vi "Main.vi"() -> ()   [LabVIEW 2014]
uses:
  Tab Panel Data.ctl
  Panel Data.ctl
  Panel Move Modes.ctl
  <vilib>/Utility/miscctls.llb/LVPoint32TypeDef.ctl
  Panel Global Methods.ctl
  <vilib>/Utility/miscctls.llb/LVPositionTypeDef.ctl
  Sub Function/Windows Utilities/WinUtil HWND/Window Style/Get Window GWL_Style.vi
  Sub Function/Windows Utilities/WinUtil HWND/Window Style/Set Window GWL_Style.vi
  Sub Function/Windows Utilities/WinUtil HWND/Get Window HWnd.vi
  Sub Function/Windows Utilities/WinUtil HWND/Get Window Rectangle (hwnd).vi
  <vilib>/Utility/inputDevices.llb/mouseAcquire.vi
  <vilib>/Utility/inputDevices.llb/closeMouse.vi
  <vilib>/Utility/cursorutil.llb/Set Cursor (Icon Pict).vi
  <userlib>/_OpenG.lib/array/array.llb/Conditional Auto-Indexing Tunnel (VI-REF)__ogtk.vi
  Sub Function/Windows Utilities/WinUtil HWND/Window Style/Modify Window Style.vi
  <userlib>/_OpenG.lib/error/error.llb/Build Error Cluster__ogtk.vi
  <vilib>/picture/picture.llb/Draw True-Color Pixmap.vi
panel:
  in  "New Tab":bool
  in  "Tab Control":T1(tab)=enum."Tab 20"
  in  "Move Panel":bool
  in  "Lock Move":bool
  in  "Add":bool
  out "error out":errorcluster
  in  "error in (no error)":errorcluster
  out "2D Picture":picture
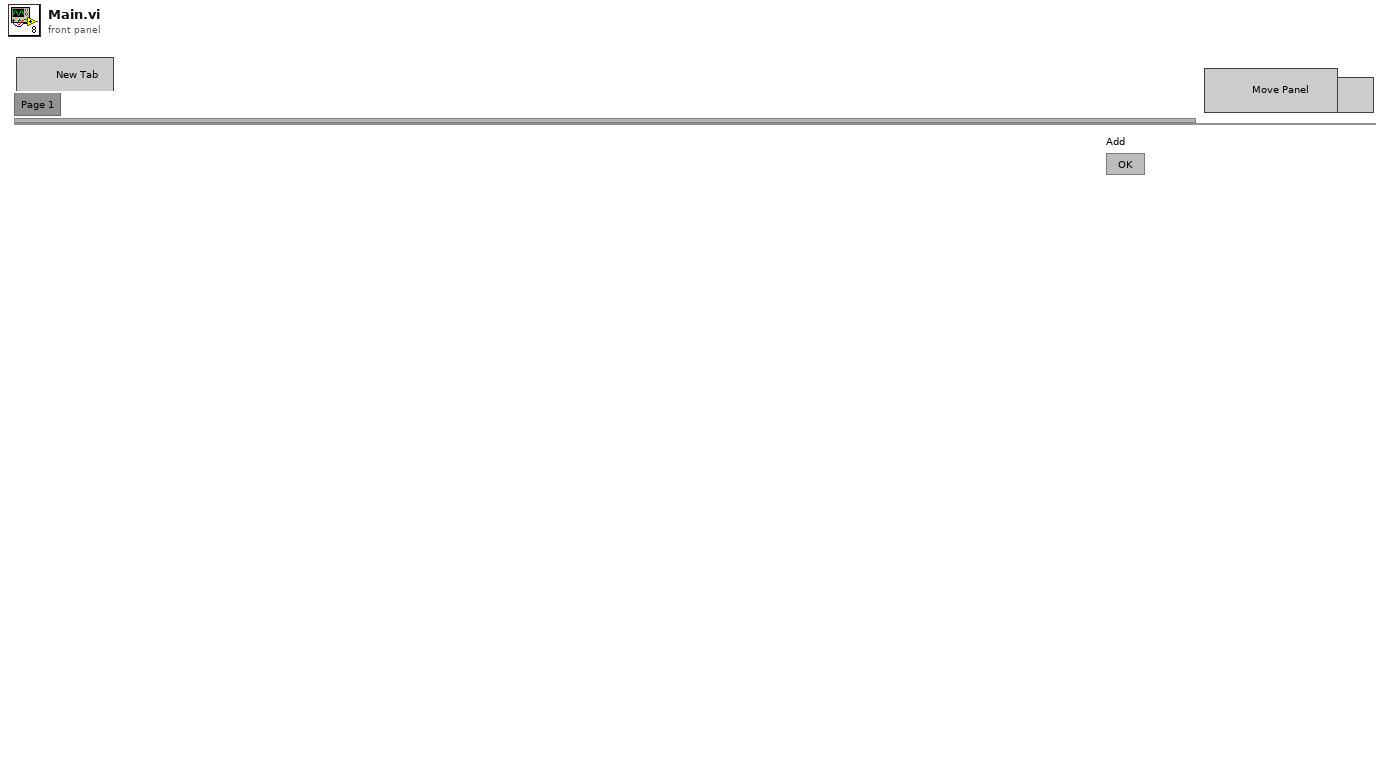
[diagram p1: front panel]
types:
  T1 = enum32{"Tab 1", "Tab 2", "Tab 3", "Tab 4", "Tab 5", "Tab 6", "Tab 7", "Tab 8", "Tab 9", "Tab 10", "Tab 11", "Tab 12", "Tab 13", "Tab 14", "Tab 15", "Tab 16", "Tab 17", "Tab 18", "Tab 19", "Tab 20"}
  T2 = typedef "LVPoint32TypeDef.ctl" = cluster{"Horizontal":i32, "Vertical":i32}
  T3 = typedef "Panel Move Modes.ctl" = enum16{"Move Off", "Move Single", "Move Locked"}
  T4 = typedef "Panel Data.ctl" = cluster{"Panel VI Name":string, "Hwnd":u32, "Collapsed?":bool, "Panel Ref":refnum<vi>, "Events Variant":variant, "Resizeable?":bool, "Un-Dockedable?":bool, "Docked?":bool}
  T5 = typedef "Tab Panel Data.ctl" = cluster{"Tab Name":string, "Tab Visible":bool, "Panel Names":string[]}
  T6 = cluster{"Event Ref":refnum<event-registration>, "New Panel VI Name":string, "Quit Event":refnum<user-event>, "Move Event":refnum<user-event>, "Dock Event":refnum<user-event>, "Panel Move Mode":T3, "Current Panel":T4, "Current Tab":i32, "Previous Tab":i32, "Reposition Offset":cluster{"Left":i16, "Top":i32}, "All Panel Data":T5[], "Parent Hwnd":u32, "Last Mouse Coor Move":T2, "Mouse Down Move":bool, "Handle Resize":bool, "Tab Mouse Coordinates":T2, "Tab Mouse Time":u32, "New Tab Mouse":bool, "Dock Panel In New Tab":bool}
  T7 = typedef "Panel Global Methods.ctl" = enum16{"Read All Panels", "Read Panel Data", "Write Panel Data"}
  T8 = enum8{"Enabled", "Disabled", "Disabled and Grayed Out"}
  T9 = enum32{"Invalid", "Standard", "Closed", "Hidden", "Minimized", "Maximized"}
  T10 = typedef "LVPositionTypeDef.ctl" = cluster{"Left":i32, "Top":i32}
  T11 = cluster{"Width":i16, "Style":enum32{"Solid", "Dash", "Dot", "DashDot", "DashDotDot"}}
  T12 = cluster{"left":i16, "top":i16, "right":i16, "bottom":i16}
  T13 = enum16{"Clear Error And Continue", "Notify User Clear Error", "Clear Error Cleanup"}
  T14 = cluster{"Horizontal":i32, "Vertical":i32, "Scrolling":i32}
  T15 = typedef "lveventtype.ctl" = enum32{"Null", "Timeout", "Annotation Menu Selection", "Annotation Menu Selection?", "App Instance Close", "App Instance Close?", "Autoscale Range Change", "Bookmark Info Change", "Cell Edit", "Cell Edit?", "Cursor Grab", "Cursor Grab?", "Cursor Menu Selection", "Cursor Menu Selection?", "Cursor Move", "Cursor Release", "Data Change", "Direction Change", "Display State Change", "Drag Ended", "Drag Enter", "Drag Leave", "Drag Over", "Drag Source Update", "Drag Starting", "Drag Starting?", "Drop", "Exec State Change", "Key Down", "Key Down?", "Key Repeat", "Key Repeat?", "Key Up", "Listbox Double Click", "Menu Activation?", "Menu Selection (App)", "Menu Selection? (App)", "Menu Selection (User)", "Mouse Down", "Mouse Down?", "Mouse Enter", "Mouse Leave", "Mouse Move", "Mouse Up", "Mouse Wheel", "NI Security User Change (App)", "Pane Size", "Panel Close", "Panel Close?", "Panel Resize", "Plot Attribute Change", "Scale Range Change", "Shortcut Menu Activation?", "Shortcut Menu Selection (App)", "Shortcut Menu Selection? (App)", "Shortcut Menu Selection (User)", "Tree Double Click", "Tree Drag", "Tree Drag?", "Tree Drop", "Tree Drop?", "Tree Item Close", "Tree Item Close?", "Tree Item Open", "Tree Item Open?", "User Event", "Value Change"}
  T16 = typedef "LVRectTypeDef.ctl" = cluster{"Left":i16, "Top":i16, "Right":i16, "Bottom":i16}
  T17 = typedef "LVBoundsTypeDef.ctl" = cluster{"Width":u32, "Height":u32}
  T18 = typedef "Window Rectangle (hwnd).ctl" = cluster{"left":i16, "top":i16, "right":i16, "bottom":i16}
  T19 = typedef "LVPointTypeDef.ctl" = cluster{"Horizontal":i16, "Vertical":i16}
  T20 = typedef "imagedata.ctl" = cluster{"image type":i32, "image depth":i32, "image":u8[], "mask":u8[], "colors":u32[], "Rectangle":cluster{"left":i16, "top":i16, "right":i16, "bottom":i16}}
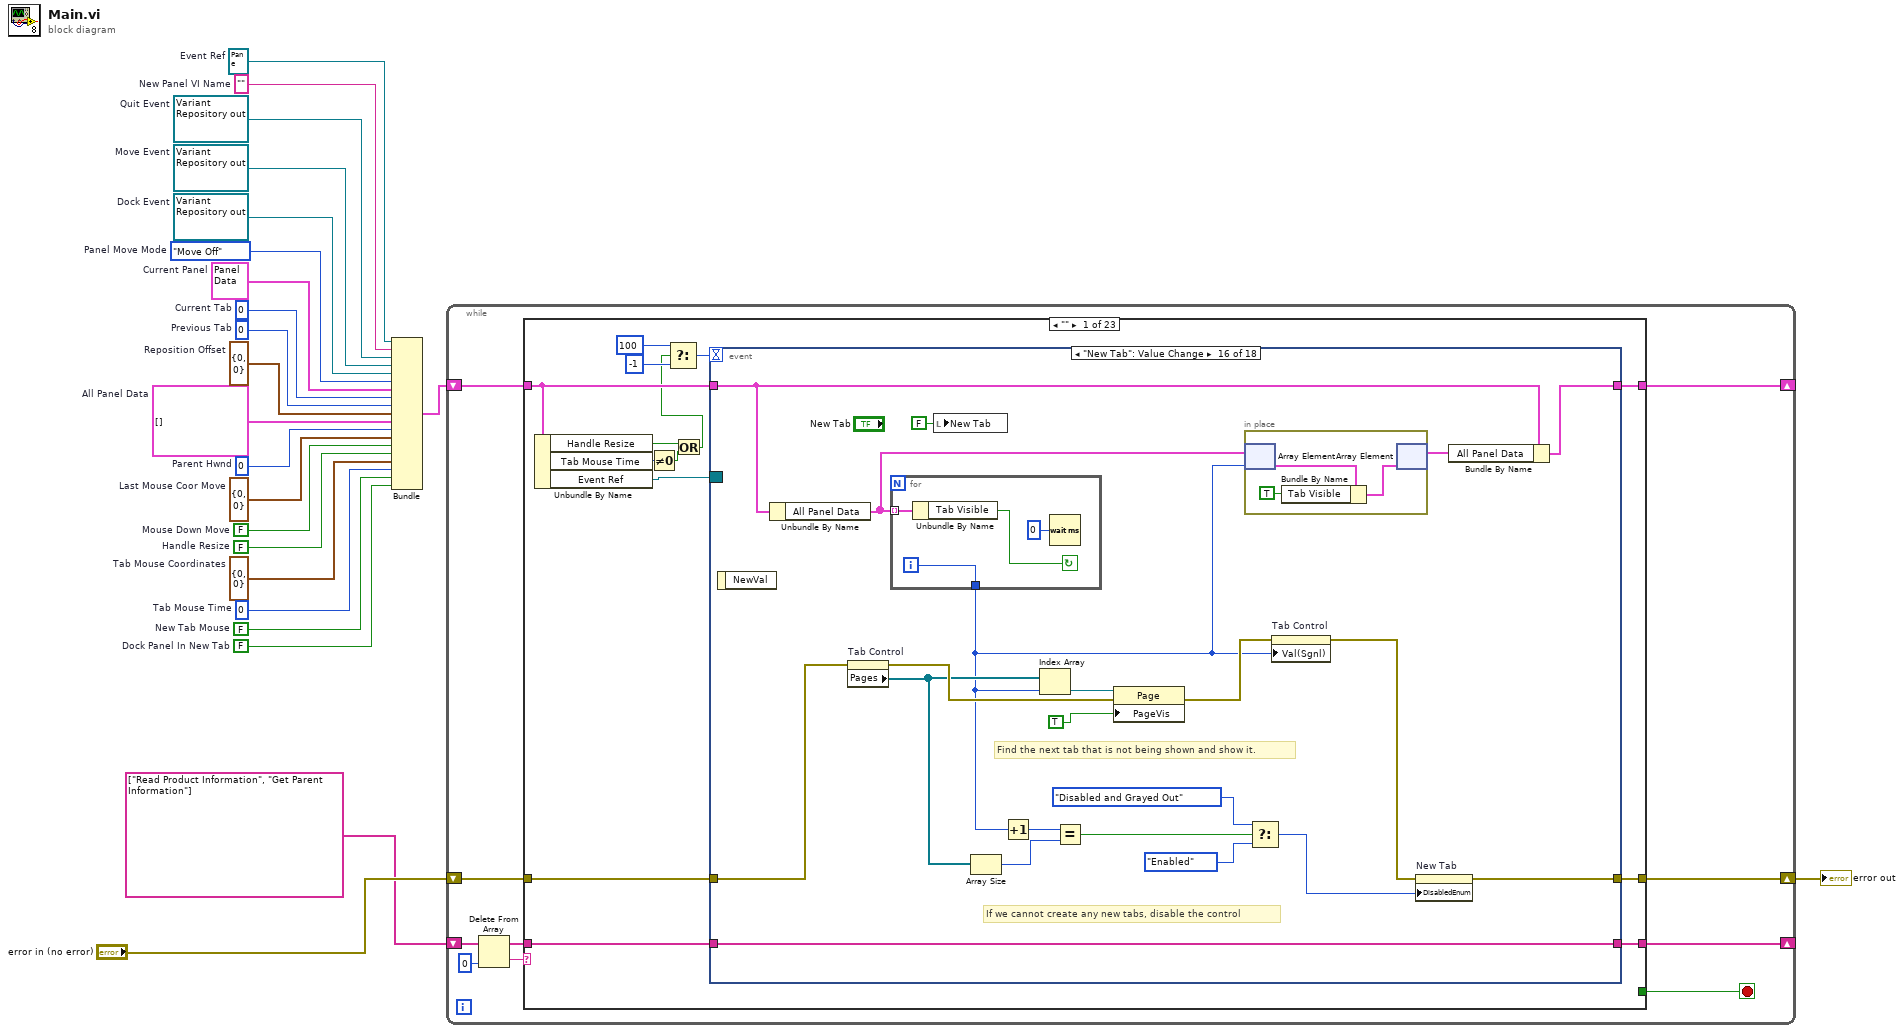
[diagram p0: block diagram]
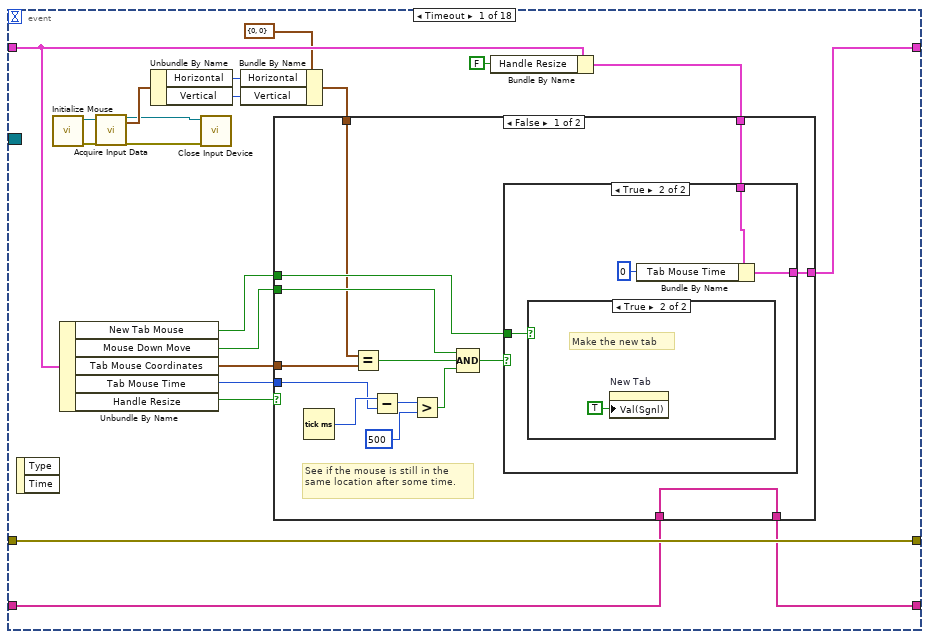
[diagram p2: hidden frame]
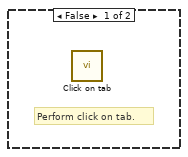
[diagram p4: hidden frame]
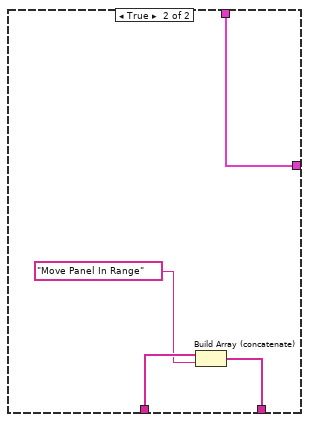
[diagram p5: hidden frame]
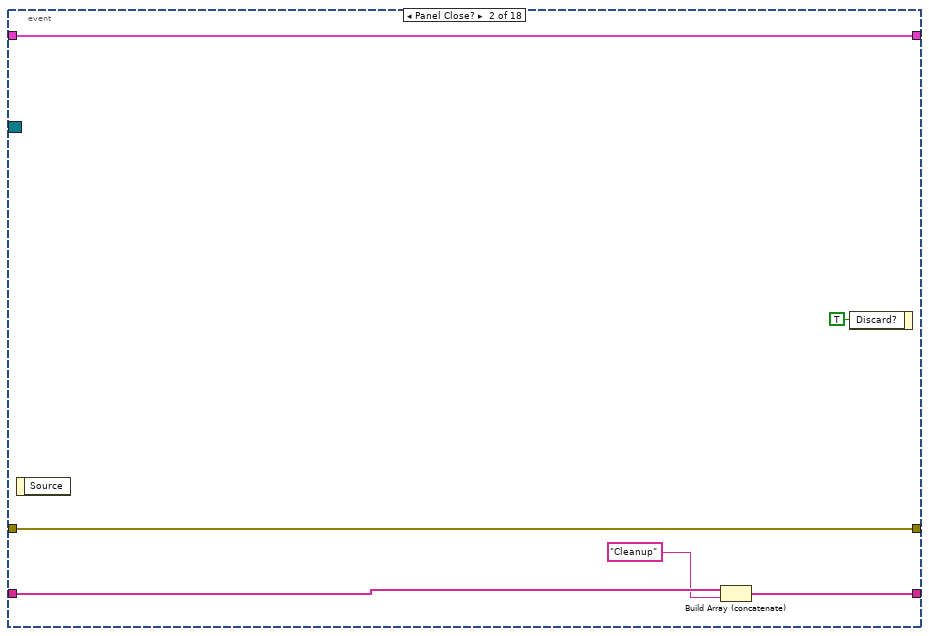
[diagram p6: hidden frame]
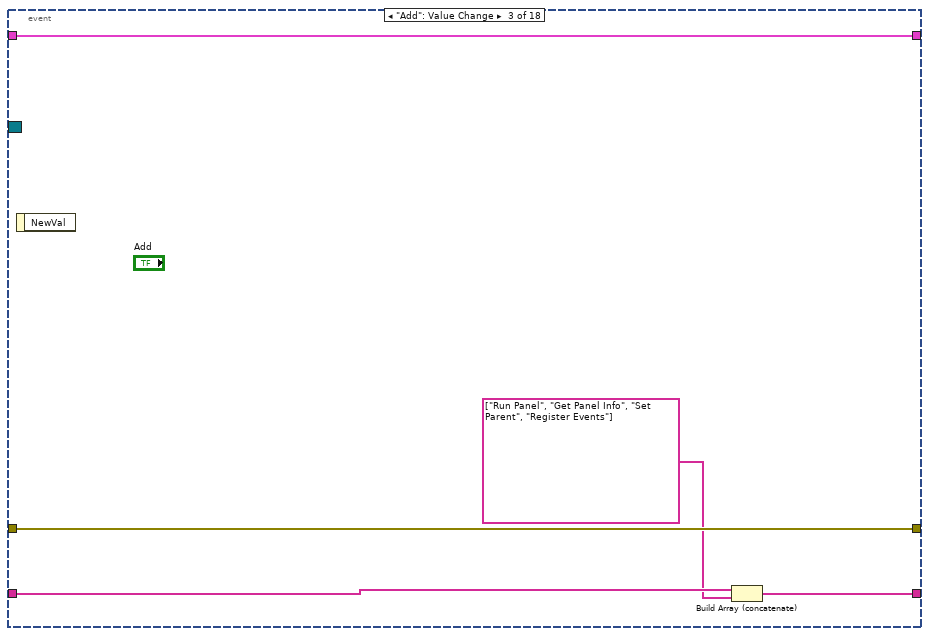
[diagram p7: hidden frame]
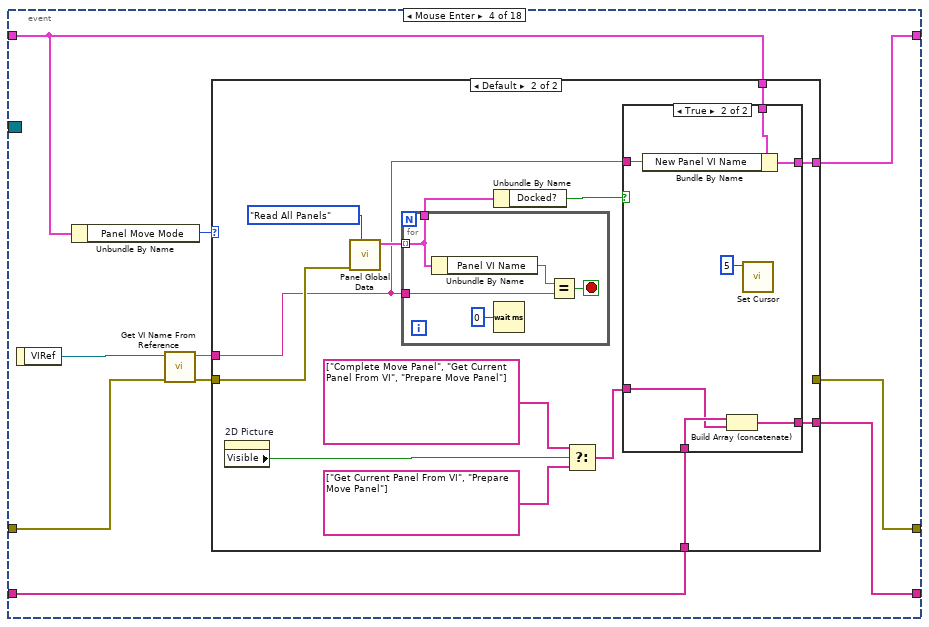
[diagram p8: hidden frame]
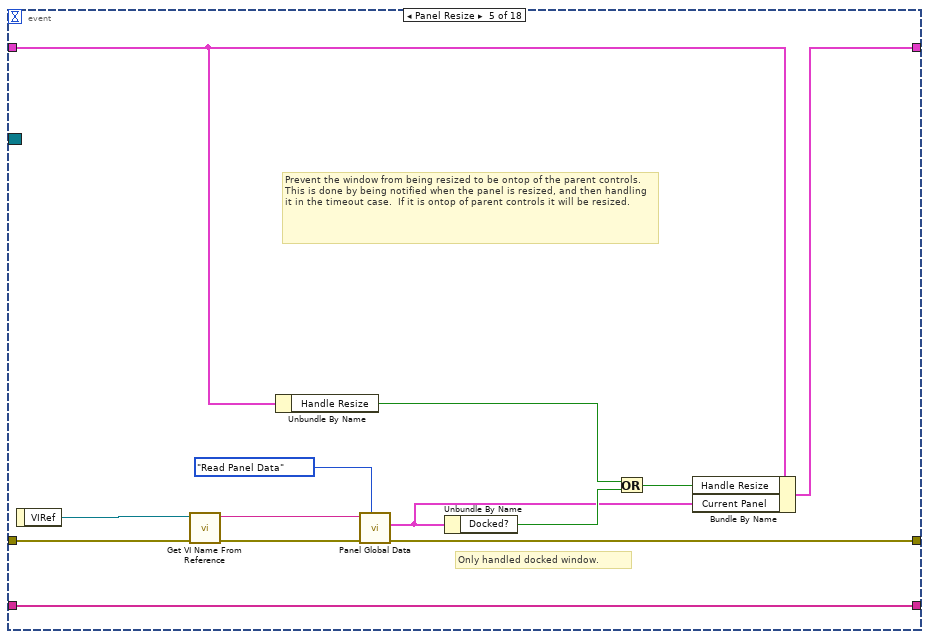
[diagram p11: hidden frame]
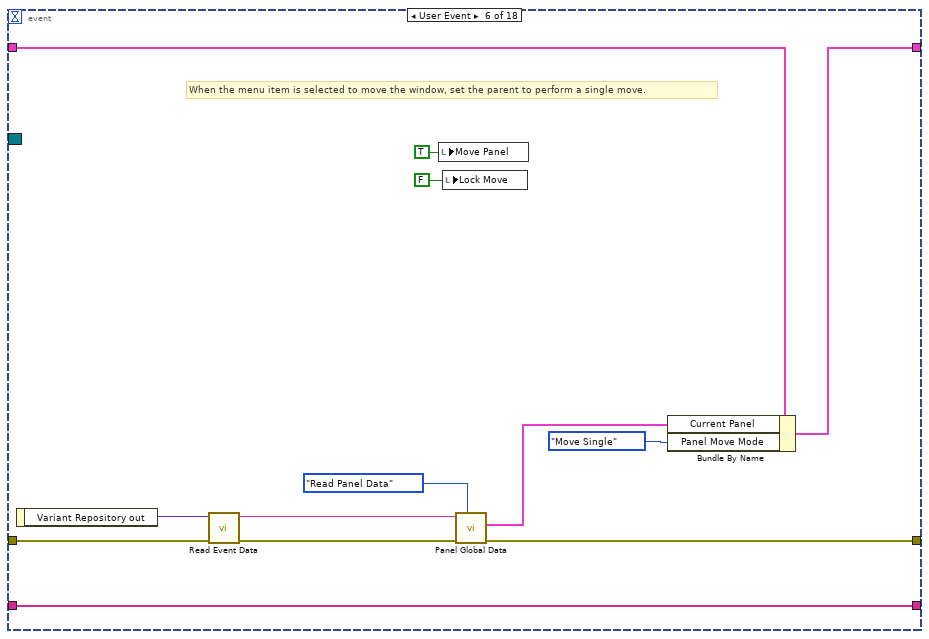
[diagram p12: hidden frame]
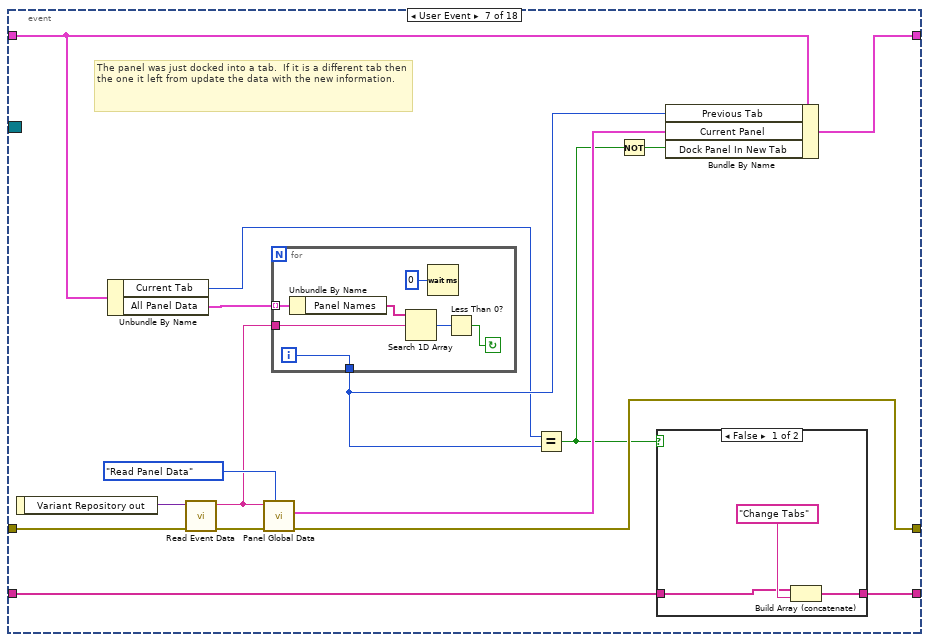
[diagram p13: hidden frame]
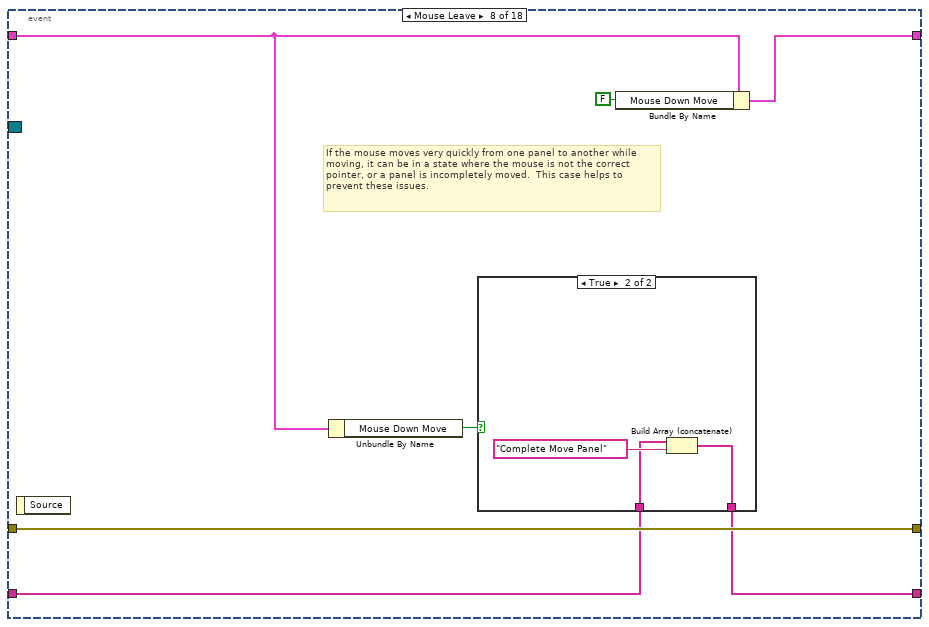
[diagram p15: hidden frame]
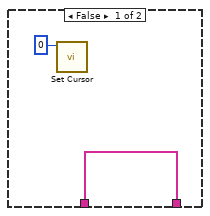
[diagram p16: hidden frame]
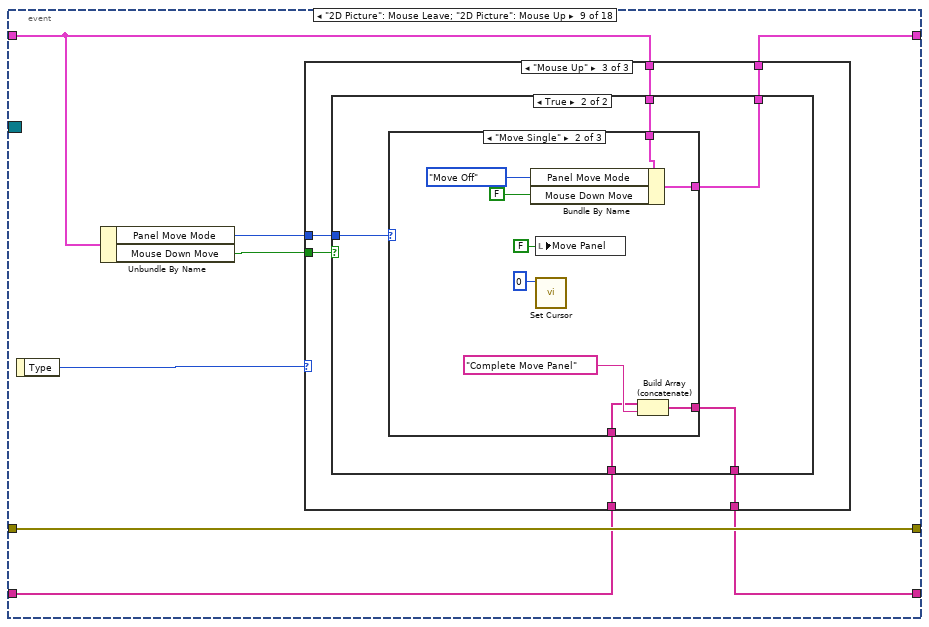
[diagram p17: hidden frame]
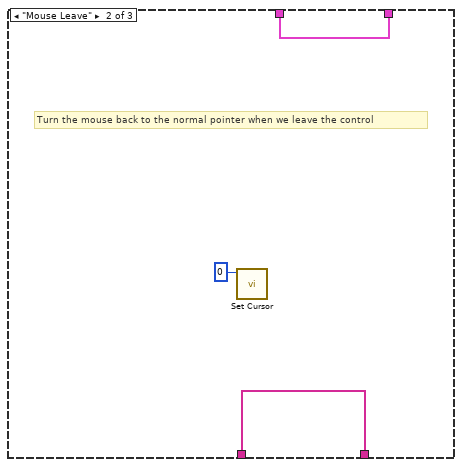
[diagram p19: hidden frame]
diagram:
  w3 = refnum<event-registration> refnum  # Event Ref
  w4 = refnum<user-event> refnum  # Quit Event
  w5 = FALSE  # Dock Panel In New Tab
  w6 = refnum<user-event> refnum  # Dock Event
  w7 = ""  # New Panel VI Name
  w8 = 0  # Previous Tab
  w9 = FALSE  # New Tab Mouse
  w10 = u32 0  # Tab Mouse Time
  w11 = T2 {"Horizontal"=0, "Vertical"=0}  # Tab Mouse Coordinates
  w12 = FALSE  # Handle Resize
  w13 = refnum<user-event> refnum  # Move Event
  w14 = FALSE  # Mouse Down Move
  w15 = T2 {"Horizontal"=0, "Vertical"=0}  # Last Mouse Coor Move
  w16 = u32 0  # Parent Hwnd
  w19 = Panel_Move_Modes."Move Off"  # Panel Move Mode
  w20 = T4 {"Panel VI Name"="", "Hwnd"=0, "Collapsed?"=FALSE, "Panel Ref"=refnum, "Events Variant"=variant, "Resizeable?"=FALSE, "Un-Dockedable?"=FALSE, "Docked?"=FALSE}  # Current Panel
  w21 = 0  # Current Tab
  w17 = T5[] []  # All Panel Data
  w18 = cluster{"Left":i16, "Top":i32} {"Left"=0, "Top"=0}  # Reposition Offset
  n1 = Bundle("Event Ref"=w3, "New Panel VI Name"=w7, "Quit Event"=w4, "Move Event"=w13, "Dock Event"=w6, "Panel Move Mode"=w19, "Current Panel"=w20, "Current Tab"=w21, "Previous Tab"=w8, "Reposition Offset"=w18, "All Panel Data"=w17, "Parent Hwnd"=w16, "Last Mouse Coor Move"=w15, "Mouse Down Move"=w14, "Handle Resize"=w12, "Tab Mouse Coordinates"=w11, "Tab Mouse Time"=w10, "New Tab Mouse"=w9, "Dock Panel In New Tab"=w5) -> (w23:T6)  [unwired: 1 in]
  n2 = while {
    shift-right: [w24] -> _
    shift-left: string[] ["Read Product Information", "Get Parent Information"] ("Initialized States") -> [w27]
    shift-right: [w29] -> w1
    shift-left: "error in (no error)" -> [w33]
    shift-right: [w31] -> _
    shift-left: w23 -> [w32]
    stop <- w30 stop-if-true
    n3 = Delete From Array(array=w27, index=0) -> (deleted portion=w25:string, array with subset deleted=w26:string[])  [unwired: 1 in]
    n4 = case "State Machine" shown="\"\"" w25 {
      selector: w25 -> [_ _ _ _ _ _ _ _ _ _ _ _ w592 _ _ _ _ w731 _ _ _ _ _]
      tunnel: w26 -> [w47 w402 w406 w447 w486 w506 w528 w555 w558 w561 w564 w573 w606 w656 w678 w709 w711 w735 w738 w741 w758 w771 w775]
      tunnel: [w43 w402 w406 w447 w486 w506 w528 w555 w558 w561 w564 w573 w606 w656 w678 w709 w712 w735 w738 w739 w758 w771 w775] -> w24
      tunnel: [w44 w400 w405 w423 w482 w497 w521 w537 w556 w559 w563 w565 w579 w651 w658 w708 w713 w728 w737 w743 w746 w769 w772] -> w29
      tunnel: w33 -> [w45 w400 w405 w417 w470 w494 w515 w542 w556 w559 w563 w566 w580 w650 w663 w708 w714 w729 w737 w743 w752 w770 w772]
      tunnel: w32 -> [w42 w401 w403 w440 w484 w502 w527 w549 w557 w560 w562 w570 w591 w652 w667 w707 w715 w734 w736 w742 w757 w768 w774]
      tunnel: [w46 w401 w403 w443 w485 w503 w522 w541 w557 w560 w562 w568 w591 w652 w662 w707 w715 w734 w736 w742 w757 w768 w774] -> w31
      tunnel: [_ _ _ _ _ _ _ _ _ _ _ _ _ _ _ _ _ _ _ _ _ _ TRUE] -> w30
      frame "" {
        n5 = Unbundle By Name(w42) -> ("Handle Resize"=w35:bool, "Tab Mouse Time"=w37:u32, "Event Ref"=w41:refnum<event-registration>)
        n6 = Not Equal To 0?(x=w37) -> (x != 0?=w36:bool)
        n7 = Or(x=w35, y=w36) -> (x .or. y?=w34:bool)
        n8 = Select(t=100, s=w34, f=-1) -> (s? t:f=w38:i32)
        n9 = event shown="[15] \"New Tab\": Value Change" {
          selector: w41 -> [_ _ _ _ _ _ _ _ _ _ _ _ _ _ _ _ _ _]
          dyn-events: _ -> [_ _ _ _ _ _ _ _ _ _ _ _ _ _ _ _ _ _]
          timeout: w38 -> [_ _ _ _ _ _ _ _ _ _ _ _ _ _ _ _ _ _]
          tunnel: w42 -> [w66 w96 w103 w110 w147 w170 w181 w201 w213 w257 w263 w276 w283 w325 w333 w353 w368 w372]
          tunnel: w47 -> [w67 w95 w101 w108 w157 w163 w186 w203 w215 w256 w269 w278 w281 w324 w327 w354 w366 w374]
          tunnel: [w59 w96 w103 w109 w156 w168 w183 w199 w212 w257 w262 w275 w290 w323 w331 w348 w368 w371] -> w46
          tunnel: w45 -> [w68 w97 w102 w105 w150 w160 w171 w204 w217 w254 w259 w279 w291 w309 w332 w345 w367 w375]
          tunnel: [w68 w97 w102 w104 w149 w162 w177 w204 w217 w253 w258 w279 w291 w308 w332 w338 w367 w375] -> w44
          tunnel: [w64 w93 w99 w107 w157 w163 w184 w202 w214 w256 w269 w278 w280 w324 w326 w354 w366 w374] -> w43
          event Timeout {
            n10 = event-data() -> ()  [unwired: 1 in, 2 out]
            n11 = call <vilib>:"Initialize Mouse.vi"() -> ("error out"=w52:errorcluster, "device ID"=w49:refnum<k1>)  [unwired: 10 in]
            n12 = Unbundle By Name(w66) -> ("New Tab Mouse"=w57:bool, "Mouse Down Move"=w58:bool, "Tab Mouse Coordinates"=w62:T2, "Tab Mouse Time"=w61:u32, "Handle Resize"=w63:bool)
            n13 = call-poly <vilib>:"Acquire Input Data.vi"("device ID"=w49, "error in (no error)"=w52) -> ("device ID"=w50:refnum<k1>, "axis info"=w53:T14, "error out"=w51:errorcluster)  [unwired: 14 in, 1 out]
            n14 = Unbundle By Name(w53) -> ("Horizontal"=w55:i32, "Vertical"=w56:i32)
            n15 = call-poly <vilib>:"Close Input Device.vi"("error in (no error)"=w51, "device ID"=w50) -> ()  [unwired: 8 in, 1 out]
            n16 = Bundle By Name(cluster=cluster{"Horizontal":i32, "Vertical":i32} {"Horizontal"=0, "Vertical"=0} ("Mouse Position"), "Horizontal"=w55, "Vertical"=w56) -> (w48:cluster{"Horizontal":i32, "Vertical":i32})
            n17 = Bundle By Name(cluster=w66, "Handle Resize"=FALSE) -> (w60:T6)
            n18 = case shown="False" w63 {
              tunnel: w67 -> [w72 w91]
              tunnel: [w72 w89] -> w64
              tunnel: w62 -> [w82 _]
              tunnel: w61 -> [w80 _]
              tunnel: w60 -> [w74 w92]
              tunnel: [w73 w92] -> w59
              tunnel: w58 -> [w71 _]
              tunnel: w57 -> [w70 _]
              tunnel: w48 -> [w69 _]
              frame False {
                # "See if the mouse is still in the same location after some time."
                n19 = Tick Count (ms)() -> (millisecond timer value=w81:u32)
                n20 = Equal?(x=w69, y=w82) -> (x = y?=w77:bool)
                n21 = Subtract(x=w81, y=w80) -> (x-y=w79:u32)
                n22 = Greater?(x=w79, y=u32 500) -> (0:w76:bool)
                n23 = Compound Arithmetic op=AND(w71, w77, w76) -> (w75:bool)
                n24 = case shown="True" w75 {
                  tunnel: w74 -> [w83 w87]
                  tunnel: [w83 w85] -> w73
                  tunnel: w70 -> [_ w84]
                  frame False {
                  }
                  frame True {
                    n25 = case shown="True" w84 {
                      frame False {
                        # "Perform click on tab."
                        n26 = call "Click on tab.vi"() -> ()  [unwired: 11 in, 1 out]
                      }
                      frame True {
                        # "Make the new tab"
                        n27 = property on="New Tab" class="Bool (strict)"("Val(Sgnl)"=TRUE ("Value (Signaling)")) -> ()  [unwired: 2 in, 2 out]
                      }
                    }
                    n28 = Bundle By Name(cluster=w87, "Tab Mouse Time"=u32 0) -> (w85:T6)
                  }
                }
              }
              frame True {
                n29 = Build Array (concatenate)(w91, "Move Panel In Range" ("String")) -> (w89:string[])
              }
            }
          }
          event Panel Close? {
            n30 = event-data() -> ()  [unwired: 1 in, 1 out]
            n31 = Build Array (concatenate)(w95, "Cleanup" ("Panel Close Event")) -> (w93:string[])
            n32 = event-data("Discard?"=TRUE) -> ()  [unwired: 1 in, 1 out]
          }
          event "Add": Value Change {
            n33 = event-data() -> ()  [unwired: 1 in, 1 out]
            n34 = Build Array (concatenate)(w101, string[] ["Run Panel", "Get Panel Info", "Set Parent", "Register Events"] ("Elements to Add")) -> (w99:string[])
          }
          event Mouse Enter {
            n35 = event-data() -> ("VIRef"=w112:refnum<vi>)  [unwired: 1 in]
            n36 = Unbundle By Name(w110) -> ("Panel Move Mode"=w113:T3)
            n37 = call "Get VI Name From Reference.vi"("error in (no error)"=w105, "VI Ref"=w112) -> ("error out"=w106:errorcluster, "VI Name"=w111:string)  [unwired: 8 in]
            n38 = case shown="Default" w113 {
              tunnel: w111 -> [_ w121]
              tunnel: w110 -> [w116 w125]
              tunnel: [w116 w124] -> w109
              tunnel: w108 -> [w115 w130]
              tunnel: [w115 w129] -> w107
              tunnel: w106 -> [w114 w122]
              tunnel: [w114 _] -> w104
              frame "Move Off" {
              }
              frame Default {
                n39 = property on="2D Picture" class="Pict"() -> ("Visible"=w117:bool)  [unwired: 2 in, 2 out]
                n40 = call "Panel Global Data.vi"("Method (Read All)"=Panel_Global_Methods."Read All Panels", "error in (no error)"=w122) -> ("All Panel Data"=w127:T4[])  [unwired: 6 in, 3 out]
                n41 = for {
                  tunnel: w121 -> [w143]
                  tunnel: [w140] -> w123
                  tunnel: w127 -> [w140] mode=indexing
                  stop <- w142 stop-if-true
                  n42 = Unbundle By Name(w140) -> ("Panel VI Name"=w144:string)
                  n43 = Wait (ms)(milliseconds to wait=u32 0) -> ()  [unwired: 1 out]
                  n44 = Equal?(x=w144, y=w143) -> (x = y?=w142:bool)
                }
                n45 = Unbundle By Name(w123) -> ("Docked?"=w126:bool)
                n46 = Select(t=string[] ["Complete Move Panel", "Get Current Panel From VI", "Prepare Move Panel"], s=w117, f=string[] ["Get Current Panel From VI", "Prepare Move Panel"]) -> (s? t:f=w118:string[])
                n47 = case shown="True" w126 {
                  tunnel: w130 -> [w132 w135]
                  tunnel: [w132 w133] -> w129
                  tunnel: w125 -> [w131 w138]
                  tunnel: [w131 w137] -> w124
                  tunnel: w118 -> [_ w134]
                  tunnel: w121 -> [_ w136]
                  frame False {
                  }
                  frame True {
                    n48 = Bundle By Name(cluster=w138, "New Panel VI Name"=w136) -> (w137:T6)
                    n49 = Build Array (concatenate)(w135, w134) -> (w133:string[])
                    n50 = call-poly <vilib>:"Set Cursor.vi"("icon"=u16 5) -> ()  [unwired: 9 in, 2 out]
                  }
                }
              }
            }
          }
          event Panel Resize {
            # "Only handled docked window."
            # "Prevent the window from being resized to be ontop of the parent controls.  This is done by being notified when the panel is resized, and then handling it in the timeout case.  If it is ontop of parent controls it will be resized."
            n51 = event-data() -> ("VIRef"=w152:refnum<vi>)  [unwired: 1 in]
            n52 = call "Get VI Name From Reference.vi"("error in (no error)"=w150, "VI Ref"=w152) -> ("error out"=w153:errorcluster, "VI Name"=w154:string)  [unwired: 8 in]
            n53 = Unbundle By Name(w147) -> ("Handle Resize"=w146:bool)
            n54 = call "Panel Global Data.vi"("Method (Read All)"=Panel_Global_Methods."Read Panel Data", "error in (no error)"=w153, "Panel VI Name"=w154) -> ("error out"=w149:errorcluster, "Panel Data Out"=w148:T4)  [unwired: 5 in, 2 out]
            n55 = Unbundle By Name(w148) -> ("Docked?"=w151:bool)
            n56 = Or(x=w146, y=w151) -> (x .or. y?=w145:bool)
            n57 = Bundle By Name(cluster=w147, "Handle Resize"=w145, "Current Panel"=w148) -> (w156:T6)
          }
          event User Event {
            # "When the menu item is selected to move the window, set the parent to perform a single move."
            n58 = event-data() -> ("Variant Repository out"=w161:variant)  [unwired: 1 in]
            n59 = call "Read Event Data.vi"("error in (no error)"=w160, "Variant Data"=w161) -> ("error out"=w158:errorcluster, "Event Name"=w159:string)  [unwired: 7 in, 1 out]
            n60 = local write "Move Panel"(TRUE ("Move Panel")) -> ()
            n61 = local write "Lock Move"(FALSE ("Lock Move")) -> ()
            n62 = call "Panel Global Data.vi"("Method (Read All)"=Panel_Global_Methods."Read Panel Data", "error in (no error)"=w158, "Panel VI Name"=w159) -> ("error out"=w162:errorcluster, "Panel Data Out"=w167:T4)  [unwired: 5 in, 2 out]
            n63 = Bundle By Name(cluster=w170, "Current Panel"=w167, "Panel Move Mode"=Panel_Move_Modes."Move Single") -> (w168:T6)
          }
          event User Event {
            # "The panel was just docked into a tab.  If it is a different tab then the one it left from update the data with the new information."
            n64 = event-data() -> ("Variant Repository out"=w174:variant)  [unwired: 1 in]
            n65 = Unbundle By Name(w181) -> ("Current Tab"=w178:i32, "All Panel Data"=w180:T5[])
            n66 = call "Read Event Data.vi"("error in (no error)"=w171, "Variant Data"=w174) -> ("error out"=w172:errorcluster, "Event Name"=w173:string)  [unwired: 7 in, 1 out]
            n67 = call "Panel Global Data.vi"("Method (Read All)"=Panel_Global_Methods."Read Panel Data", "error in (no error)"=w172, "Panel VI Name"=w173) -> ("error out"=w177:errorcluster, "Panel Data Out"=w182:T4)  [unwired: 5 in, 2 out]
            n68 = for {
              tunnel: w180 -> [w197] mode=indexing
              tunnel: w173 -> [w195]
              tunnel: [w191] -> w179
              i -> [w191]
              stop <- w193 continue-if-true
              n69 = Unbundle By Name(w197) -> ("Panel Names"=w196:string[])
              n70 = Search 1D Array(1D array=w196, element=w195) -> (index of element=w194:i32)  [unwired: 1 in]
              n71 = Wait (ms)(milliseconds to wait=u32 0) -> ()  [unwired: 1 out]
              n72 = Less Than 0?(x=w194) -> (x < 0?=w193:bool)
            }
            n73 = Equal?(x=w178, y=w179) -> (x = y?=w176:bool)
            n74 = Not(x=w176) -> (.not. x?=w175:bool)
            n75 = case shown="False" w176 {
              tunnel: w186 -> [w188 w190]
              tunnel: [w187 w190] -> w184
              frame False {
                n76 = Build Array (concatenate)(w188, "Change Tabs" ("String")) -> (w187:string[])
              }
              frame True {
                # "Tab did not change."
              }
            }
            n77 = Bundle By Name(cluster=w181, "Previous Tab"=w179, "Current Panel"=w182, "Dock Panel In New Tab"=w175) -> (w183:T6)
          }
          event Mouse Leave {
            # "If the mouse moves very quickly from one panel to another while moving, it can be in a state where the mouse is not the correct pointer, or a panel is incompletely moved.  This case helps to prevent these issues."
            n78 = event-data() -> ()  [unwired: 1 in, 1 out]
            n79 = Unbundle By Name(w201) -> ("Mouse Down Move"=w200:bool)
            n80 = case shown="True" w200 {
              tunnel: w203 -> [w206 w208]
              tunnel: [w206 w207] -> w202
              frame False {
                n81 = call-poly <vilib>:"Set Cursor.vi"("icon"=u16 0) -> ()  [unwired: 9 in, 2 out]
              }
              frame True {
                n82 = Build Array (concatenate)(w208, "Complete Move Panel" ("String")) -> (w207:string[])
              }
            }
            n83 = Bundle By Name(cluster=w201, "Mouse Down Move"=FALSE) -> (w199:T6)
          }
          event "2D Picture": Mouse Leave; "2D Picture": Mouse Up {
            n84 = event-data() -> ("Type"=w210:T15)  [unwired: 1 in]
            n85 = Unbundle By Name(w213) -> ("Panel Move Mode"=w216:T3, "Mouse Down Move"=w211:bool)
            n86 = case shown="\"Mouse Up\"" w210 {
              tunnel: w216 -> [_ _ w228]
              tunnel: w215 -> [w219 w220 w227]
              tunnel: [w219 w220 w226] -> w214
              tunnel: w213 -> [w218 w222 w225]
              tunnel: [w218 w222 w224] -> w212
              tunnel: w211 -> [_ _ w223]
              frame "Null", Default {
              }
              frame "Mouse Leave" {
                # "Turn the mouse back to the normal pointer when we leave the control"
                n87 = call-poly <vilib>:"Set Cursor.vi"("icon"=u16 0) -> ()  [unwired: 9 in, 2 out]
              }
              frame "Mouse Up" {
                n88 = case shown="True" w223 {
                  tunnel: w228 -> [_ w235]
                  tunnel: w227 -> [w229 w234]
                  tunnel: [w229 w233] -> w226
                  tunnel: w225 -> [w230 w232]
                  tunnel: [w230 w231] -> w224
                  frame False {
                  }
                  frame True {
                    n89 = case shown="\"Move Single\"" w235 {
                      tunnel: w234 -> [w239 w241 w252]
                      tunnel: [w239 w240 w252] -> w233
                      tunnel: w232 -> [w238 w247 w251]
                      tunnel: [w237 w246 w250] -> w231
                      frame "Move Off" {
                        n90 = Bundle By Name(cluster=w238, "Mouse Down Move"=FALSE) -> (w237:T6)
                      }
                      frame "Move Single" {
                        n91 = Bundle By Name(cluster=w247, "Panel Move Mode"=Panel_Move_Modes."Move Off", "Mouse Down Move"=FALSE) -> (w246:T6)
                        n92 = local write "Move Panel"(FALSE ("Move Panel")) -> ()
                        n93 = call-poly <vilib>:"Set Cursor.vi"("icon"=u16 0) -> ()  [unwired: 9 in, 2 out]
                        n94 = Build Array (concatenate)(w241, "Complete Move Panel" ("String")) -> (w240:string[])
                      }
                      frame "Move Locked" {
                        n95 = Bundle By Name(cluster=w251, "Mouse Down Move"=FALSE) -> (w250:T6)
                      }
                    }
                  }
                }
              }
            }
          }
          event "2D Picture": Mouse Enter {
            # "Set the mouse to the movement cursor."
            n96 = event-data() -> ()  [unwired: 1 in, 3 out]
            n97 = call-poly <vilib>:"Set Cursor.vi"("error in (no error)"=w254, "icon"=u16 5) -> ("error out"=w253:errorcluster)  [unwired: 8 in, 1 out]
          }
          event "2D Picture": Mouse Move {
            # "Calculate the difference in movement from the last time this event was generated and move the picture control the same amount."
            n98 = event-data() -> ("Coords"=w264:T2)  [unwired: 1 in]
            n99 = Unbundle By Name(w263) -> ("Mouse Down Move"=w261:bool, "Last Mouse Coor Move"=w268:T2)
            n100 = property on="2D Picture" class="Pict"(error in=w259) -> (error out=w260:errorcluster, "Position"=w266:T10)  [unwired: 1 in, 1 out]
            n101 = Subtract(x=w264, y=w268) -> (x-y=w265:T2)
            n102 = Add(x=w266, y=w265) -> (x+y=w267:T10)
            n103 = case shown="True" w261 {
              tunnel: w267 -> [_ w273]
              tunnel: w260 -> [w270 w272]
              tunnel: [w270 w271] -> w258
              frame False {
              }
              frame True {
                n104 = property on="2D Picture" class="Pict"(error in=w272, "Position"=w273) -> (error out=w271:errorcluster)  [unwired: 1 in, 1 out]
              }
            }
            n105 = Bundle By Name(cluster=w263, "Last Mouse Coor Move"=w264) -> (w262:T6)
          }
          event "2D Picture": Mouse Down {
            # "Record the cursor position so we know how to move the Panel VI."
            n106 = event-data() -> ("Coords"=w274:T2)  [unwired: 1 in]
            n107 = Bundle By Name(cluster=w276, "Mouse Down Move"=TRUE, "Last Mouse Coor Move"=w274) -> (w275:T6)
          }
          event "Move Panel", "Lock Move": Value Change {
            # "If moving is turned off then move any un complete panel."
            # "Control the Move Panel and Lock Move Panel buttons based on the value change."
            n108 = event-data() -> ("NewVal"=w284:bool)  [unwired: 1 in]
            n109 = Build Array("Move Panel", "Lock Move") -> (w287:bool[])
            n110 = Boolean Array To Number(Boolean array=w287) -> (number=w286:u32)
            n111 = case shown="False" w284 {
              tunnel: w286 -> [_ w301]
              tunnel: [Panel_Move_Modes."Move Off" ("Panel Move Mode") w300] -> w285
              tunnel: [w296 _] -> w282
              frame False {
                # "If just turned false, turn Off"
                n112 = local write "Move Panel"(FALSE ("Move Panel")) -> ()
                n113 = local write "Lock Move"(FALSE ("Move Panel")) -> ()
                n114 = property on="2D Picture" class="Pict"() -> ("Visible"=w296:bool)  [unwired: 2 in, 2 out]
              }
              frame True {
                n115 = case shown="1" w301 {
                  tunnel: [Panel_Move_Modes."Move Off" ("Panel Move Mode") Panel_Move_Modes."Move Single" ("Panel Move Mode") Panel_Move_Modes."Move Locked" ("Panel Move Mode") Panel_Move_Modes."Move Locked" ("Panel Move Mode")] -> w300
                  frame 0, Default {
                  }
                  frame 1 {
                    n116 = local write "Lock Move"(FALSE ("Lock Move")) -> ()
                  }
                  frame 2 {
                    n117 = local write "Move Panel"(TRUE ("Move Panel")) -> ()
                  }
                  frame 3 {
                  }
                }
              }
            }
            n118 = case shown="True" w282 {
              tunnel: w281 -> [w292 w295]
              tunnel: [w292 w293] -> w280
              frame False {
              }
              frame True {
                n119 = Build Array (concatenate)(w295, string[] ["Complete Move Panel"] ("Elements to Add")) -> (w293:string[])
              }
            }
            n120 = Bundle By Name(cluster=w283, "Panel Move Mode"=w285) -> (w290:T6)
          }
          event "Tab Control", "New Tab": Mouse Move {
            # "Store the position of the mouse when over the tab or new tab button.  If the mouse is still in the same location after some time (in the timeout case) we will move the panel to this tab."
            n121 = event-data() -> ("CtlRef"=w321:refnum<vi>, "Time"=w322:u32)  [unwired: 1 in]
            n122 = call <vilib>:"Initialize Mouse.vi"("error in (no error)"=w309) -> ("error out"=w314:errorcluster, "device ID"=w311:refnum<k1>)  [unwired: 9 in]
            n123 = call-poly <vilib>:"Acquire Input Data.vi"("device ID"=w311, "error in (no error)"=w314) -> ("device ID"=w312:refnum<k1>, "axis info"=w315:T14, "error out"=w313:errorcluster)  [unwired: 14 in, 1 out]
            n124 = control-ref of="New Tab"() -> (w320:refnum<vi>)
            n125 = Unbundle By Name(w315) -> ("Horizontal"=w317:i32, "Vertical"=w318:i32)
            n126 = call-poly <vilib>:"Close Input Device.vi"("error in (no error)"=w313, "device ID"=w312) -> ("error out"=w308:errorcluster)  [unwired: 8 in]
            n127 = Equal?(x=w320, y=w321) -> (x = y?=w319:bool)
            n128 = Bundle By Name(cluster=cluster{"Horizontal":i32, "Vertical":i32} {"Horizontal"=0, "Vertical"=0} ("Mouse Position"), "Horizontal"=w317, "Vertical"=w318) -> (w310:cluster{"Horizontal":i32, "Vertical":i32})
            n129 = Bundle By Name(cluster=w325, "New Tab Mouse"=w319, "Tab Mouse Time"=w322, "Tab Mouse Coordinates"=w310) -> (w323:T6)
          }
          event "Tab Control": Value Change {
            # "Change the tab that we are on."
            n130 = event-data() -> ("OldVal"=w329:T1)  [unwired: 1 in]
            n131 = Bundle By Name(cluster=w333, "Current Tab"="Tab Control", "Previous Tab"=w329) -> (w331:T6)
            n132 = Build Array (concatenate)(w327, "Change Tabs" ("String")) -> (w326:string[])
          }
          event "New Tab": Value Change {
            # "Find the next tab that is not being shown and show it."
            # "If we cannot create any new tabs, disable the control"
            n133 = event-data() -> ()  [unwired: 1 in, 1 out]
            n134 = Unbundle By Name(w353) -> ("All Panel Data"=w349:T5[])
            n135 = property on="Tab Control" class="TabCtl (strict)"(error in=w345) -> (error out=w351:errorcluster, "Pages"=w344:refnum<vi>[])  [unwired: 1 in, 1 out]
            n136 = for {
              tunnel: w349 -> [w359] mode=indexing
              tunnel: [w358] -> w342
              i -> [w358]
              stop <- w361 continue-if-true
              n137 = Unbundle By Name(w359) -> ("Tab Visible"=w361:bool)
              n138 = Wait (ms)(milliseconds to wait=u32 0) -> ()  [unwired: 1 out]
            }
            n139 = local write "New Tab"(FALSE ("New Tab")) -> ()
            n140 = Array Size(array=w344) -> (size(s)=w341:i32)
            n141 = Increment(x=w342) -> (x+1=w340:i32)
            n142 = Index Array(array=w344, index=w342) -> (element=w352:refnum<vi>)
            n143 = Equal?(x=w340, y=w341) -> (x = y?=w337:bool)
            n144 = property class="Page"(reference=w352, error in=w351, "PageVis"=TRUE ("Page Visible")) -> (error out=w350:errorcluster)  [unwired: 1 out]
            n145 = in-place {
              n146 = in-place-array #1(w349, w342) -> (w357:T5)
              n147 = Bundle By Name(cluster=w357, "Tab Visible"=TRUE) -> (w355:T5)
              n148 = in-place-array #1(w355) -> (w347:T5[])  [unwired: 1 out]
            }
            n149 = Select(t=T8."Disabled and Grayed Out" ("Disabled"), s=w337, f=T8."Enabled" ("Disabled")) -> (s? t:f=w334:T8)
            n150 = property on="Tab Control" class="TabCtl (strict)"(error in=w350, "Val(Sgnl)"=w342) -> (error out=w339:errorcluster)  [unwired: 1 in, 1 out]
            n151 = property on="New Tab" class="Bool (strict)"(error in=w339, "DisabledEnum"=w334) -> (error out=w338:errorcluster)  [unwired: 1 in, 1 out]
            n152 = Bundle By Name(cluster=w353, "All Panel Data"=w347) -> (w348:T6)
          }
          event "Tab Control": Shortcut Menu Activation? {
            n153 = event-data() -> ("MenuRef"=w365:refnum<k9>)  [unwired: 1 in]
            n154 = property on="New Tab" class="Bool (strict)"() -> ("DisabledEnum"=w364:T8)  [unwired: 2 in, 2 out]
            n155 = Equal?(x=w364, y=T8."Enabled") -> (x = y?=w362:bool)
            n156 = case shown="True" w362 {
              tunnel: w365 -> [_ w370]
              frame False {
              }
              frame True {
                n157 = Insert Menu Items(8:"New Tab", 9:w370) -> ()  [unwired: 4 in, 3 out]
              }
            }
            n158 = event-data() -> ()  [unwired: 2 in, 1 out]
          }
          event "Tab Control": Shortcut Menu Selection (User) {
            n159 = event-data() -> ("ItemTag"=w373:string)  [unwired: 1 in]
            n160 = case shown="\"Rename Tab\"" w373 {
              tunnel: w372 -> [w376 w377 w385 w399]
              tunnel: w372 -> [_ _ w384 _]
              tunnel: [w376 w377 w380 w399] -> w371
              frame Default {
              }
              frame "New Tab" {
                n161 = property on="New Tab" class="Bool (strict)"("Val(Sgnl)"=TRUE ("Value (Signaling)")) -> ()  [unwired: 2 in, 2 out]
              }
              frame "Rename Tab" {
                n162 = Unbundle By Name(w384) -> ("All Panel Data"=w383:T5[], "Current Tab"=w382:i32)
                n163 = call "Rename Tab"() -> ("Tab Name"=w381:string, "OK"=w379:bool)  [unwired: 17 in, 1 out]
                n164 = case shown="True" w379 {
                  tunnel: w385 -> [w386 w392]
                  tunnel: w383 -> [_ w391]
                  tunnel: w382 -> [_ w390]
                  tunnel: w381 -> [_ w389]
                  tunnel: [w386 w387] -> w380
                  frame False {
                  }
                  frame True {
                    n165 = in-place {
                      in-place-border: w389 -> [w397]
                      n166 = in-place-array #2(w391, w390) -> (w398:T5)
                      n167 = Bundle By Name(cluster=w398, "Tab Name"=w397) -> (w396:T5)
                      n168 = in-place-array #2(w396) -> (w388:T5[])  [unwired: 1 out]
                    }
                    n169 = property on="Tab Control" class="TabCtl (strict)"() -> (error out=w394:errorcluster, "Pages"=w393:refnum<vi>[])  [unwired: 2 in, 1 out]
                    n170 = Index Array(array=w393, index=w390) -> (element=w395:refnum<vi>)
                    n171 = property class="Page"(reference=w395, error in=w394, "TabCaption"=w389) -> ()  [unwired: 2 out]
                    n172 = Bundle By Name(cluster=w392, "All Panel Data"=w388) -> (w387:T6)
                  }
                }
              }
              frame "Remove Tab" {
              }
            }
          }
        }
      }
      frame "----Initialize----" {
      }
      frame "Read Product Information" {
        # "Read the product information and display it."
        n173 = property on="2D Picture" class="Pict"("Visible"=FALSE) -> ()  [unwired: 2 in, 2 out]
      }
      frame "Get Parent Information" {
        # "Create the place holding data for the possible tabs."
        n174 = property on="Tab Control" class="TabCtl (strict)"(error in=w417) -> (error out=w420:errorcluster, "Pages"=w424:refnum<vi>[])  [unwired: 1 in, 1 out]
        n175 = Unbundle By Name(w440) -> ("All Panel Data"=w439:T5[])
        n176 = local write "Tab Control"(T1."Tab 1" ("Tab Control")) -> ()
        n177 = Index Array(array=w439) -> (element=w438:T5)  [unwired: 1 in]
        n178 = call "Get Window Handle.vi"("error in (no error)"=w417) -> ("error out"=w416:errorcluster, "HWnd Out"=w415:u32)  [unwired: 9 in]
        n179 = control-ref of="Splitter"() -> (w441:refnum<vi>)
        n180 = for {
          tunnel: w438 -> [w463]
          tunnel: [w462] -> w437 mode=indexing
          tunnel: w424 -> [w460] mode=indexing
          shift-right: [w458] -> w414
          shift-left: w420 -> [w457]
          i -> [w452]
          n181 = Increment(x=w452) -> (x+1=w455:i32)
          n182 = Format Into String(format string="Page %d", w455) -> (resulting string=w459:string)  [unwired: 2 in, 1 out]
          n183 = Wait (ms)(milliseconds to wait=u32 0) -> ()  [unwired: 1 out]
          n184 = Equal To 0?(x=w452) -> (x = 0?=w453:bool)
          n185 = Bundle By Name(cluster=w463, "Tab Name"=w459, "Tab Visible"=w453) -> (w462:T5)
          n186 = property class="Page"(reference=w460, error in=w457, "PageVis"=w453, "IndependentLabel"=TRUE ("Independent Label"), "TabCaption"=w459) -> (error out=w458:errorcluster)  [unwired: 1 out]
        }
        n187 = property class="VI"() -> (error out=w421:errorcluster, "Panel"=w426:refnum<vi>)  [unwired: 2 in, 1 out]
        n188 = property class="Splitter"(reference=w441, error in=w416) -> (error out=w442:errorcluster, "Position"=w444:i32)  [unwired: 1 out]
        n189 = property class="Pnl"(reference=w426, error in=w421) -> ("Bounds Rect"=w431:T16)  [unwired: 2 out]
        n190 = property on="Pane 3" class="Pane"() -> ("Bounds"=w419:T17)  [unwired: 2 in, 2 out]
        n191 = Unbundle By Name(w419) -> ("Height"=w436:u32)
        n192 = Unbundle(w431) -> ("Left"=w430:i16, "Top"=w429:i16)  [unwired: 2 out]
        n193 = Bundle("Left"=w430, "Top"=w429) -> (w427:cluster{"Left":i16, "Top":i16})  [unwired: 1 in]
        n194 = Increment(x=w444) -> (x+1=w445:i32)
        n195 = Add(x=u32 2, y=w436) -> (x+y=w433:u32)
        n196 = Bundle("left"=i16 0, w445) -> ()  [unwired: 1 in, 1 out]
        n197 = Bundle("Height"=u32 0, w433) -> (w432:cluster{"Height":u32, u32})  [unwired: 1 in]
        n198 = Add(x=w427, y=w432) -> (x+y=w428:cluster{u32, u32})
        n199 = for {
          tunnel: [w450] -> w413 mode=indexing
          tunnel: string[] ["Move Window", "Dock Window"] ("User Event Names") -> [_] mode=indexing
          shift-right: [w449] -> w411
          shift-left: w414 -> [w451]
          tunnel: variant ("Event Data") -> [w448]
          n200 = Create User Event(user event datatype=w448, error in=w451) -> (user event=w450:refnum<user-event>, error out=w449:errorcluster)
        }
        n201 = Create User Event(user event datatype=variant ("Event Data"), error in=w411) -> (user event=w408:refnum<user-event>, error out=w407:errorcluster)
        n202 = Index Array(array=w413) -> (element #1=w425:refnum<user-event>, element #2=w418:refnum<user-event>)  [unwired: 2 in]
        n203 = Bundle By Name(cluster=w440, "Move Event"=w425, "Dock Event"=w418, "All Panel Data"=w437, "Reposition Offset"=w428, "Parent Hwnd"=w415, "Quit Event"=w408) -> (w443:T6)
        n204 = Merge Errors(w407, w442) -> (w423:errorcluster)
      }
      frame "Run Panel" {
        w468 = string[] ["Set Settings", "Get Settings", "Get Settings.Reply"] ("User Event Names")
        # "Run the Panel VI (which will run the Child VI)"
        n205 = Unbundle By Name(w484) -> ("Move Event"=w474:refnum<user-event>, "Dock Event"=w472:refnum<user-event>, "Quit Event"=w469:refnum<user-event>)
        n206 = property on="Pane 3" class="Pane"() -> ("Bounds"=w473:T17)  [unwired: 2 in, 2 out]
        n207 = for {
          tunnel: [w489] -> w467 mode=indexing
          shift-right: [w488] -> w466
          shift-left: w470 -> [w490]
          tunnel: variant ("Event Data") -> [w487]
          tunnel: w468 -> [_] mode=indexing
          n208 = Create User Event(user event datatype=w487, error in=w490) -> (user event=w489:refnum<user-event>, error out=w488:errorcluster)
        }
        n209 = Unbundle By Name(w473) -> ("Height"=w479:u32)
        n210 = Add(x=u32 2, y=w479) -> (x+y=w476:u32)
        n211 = control-ref of="Pane 2"() -> (w480:refnum<vi>)
        n212 = Bundle("Height"=u32 0, w476) -> (w475:cluster{"Height":u32, u32})  [unwired: 1 in]
        n213 = call "Flatten User Events to Variant.vi"("error in (no error)"=w466, "All User Events"=w467, "All User Event Names"=w468, "Quit Event"=w469) -> ("error out"=w465:errorcluster, "Variant"=w464:variant)  [unwired: 6 in]
        n214 = call "Run Panel.vi"("Dock Event"=w472, "Pane Offset"=w475, "error in (no error)"=w470, "Variant Repository Out"=w464, "Move Event"=w474, "Pane in"=w480) -> ("error out"=w483:errorcluster, "Panel VI Ref"=w481:refnum<vi>)  [unwired: 4 in]
        n215 = Bundle By Name(cluster=w484, "Current Panel.Panel Ref"=w481, "Current Panel.Events Variant"=w464) -> (w485:T6)
        n216 = Merge Errors(w483, w465) -> (w482:errorcluster)
      }
      frame "Get Panel Info" {
        n217 = Unbundle By Name(w502) -> ("All Panel Data"=w505:T5[], "Current Tab"=w504:i32, "Current Panel.Events Variant"=w499:variant, "Current Panel.Panel Ref"=w496:refnum<vi>)
        n218 = call "Get VI Name From Reference.vi"("error in (no error)"=w494, "VI Ref"=w496) -> ("error out"=w493:errorcluster, "VI Name"=w495:string)  [unwired: 8 in]
        n219 = call "Panel Global Data.vi"("Method (Read All)"=Panel_Global_Methods."Read Panel Data", "error in (no error)"=w493, "Panel VI Name"=w495) -> ("error out"=w497:errorcluster, "Panel Data Out"=w492:T4)  [unwired: 5 in, 2 out]
        n220 = Bundle By Name(cluster=w492, "Events Variant"=w499) -> (w500:T4)
        n221 = Unbundle By Name(w492) -> ("Panel VI Name"=w491:string)
        n222 = in-place {
          in-place-border: w491 -> [w508]
          n223 = in-place-array #3(w505, w504) -> (w507:T5)
          n224 = Unbundle By Name(w507) -> ("Panel Names"=w510:string[])
          n225 = Build Array (concatenate)(w510, w508) -> (w509:string[])
          n226 = Bundle By Name(cluster=w507, "Panel Names"=w509) -> (w511:T5)
          n227 = in-place-array #3(w511) -> (w501:T5[])  [unwired: 1 out]
        }
        n228 = Bundle By Name(cluster=w502, "All Panel Data"=w501, "Current Panel"=w500) -> (w503:T6)
      }
      frame "Register Events" {
        # "Only respond to the Panels that are docked.  We don't care if our mouse enters when the window is floating."
        # "Any Panel that generates the Dock or Move event we need to respond to."
        n229 = Unbundle By Name(w527) -> ("Event Ref"=w525:refnum<event-registration>, "Dock Event"=w520:refnum<user-event>, "Move Event"=w526:refnum<user-event>)
        n230 = call "Panel Global Data.vi"("Method (Read All)"=Panel_Global_Methods."Read All Panels", "error in (no error)"=w515) -> ("error out"=w514:errorcluster, "All Panel Data"=w519:T4[])  [unwired: 6 in, 2 out]
        n231 = for {
          tunnel: w519 -> [w531] mode=indexing
          tunnel: [w530] -> w516 mode=indexing
          tunnel: [w529] -> w517 mode=indexing
          n232 = Unbundle By Name(w531) -> ("Panel Ref"=w530:refnum<vi>, "Docked?"=w529:bool)
          n233 = Wait (ms)(milliseconds to wait=u32 0) -> ()  [unwired: 1 out]
        }
        n234 = Unregister For Events(event registration refnum=w525, error in=w514) -> (error out=w524:errorcluster)
        n235 = call <vilib>:"Clear Errors.vi"("error in (no error)"=w524) -> ("error out"=w523:errorcluster)  [unwired: 5 in, 1 out]
        n236 = call-poly <userlib>:"Conditional Auto-Indexing Tunnel__ogtk.vi"("Array in"=w516, "Elements to keep"=w517) -> ("Filtered Array out"=w513:refnum<vi>[])  [unwired: 5 in]
        n237 = register-events(error in=w523, w520, w526, w513, w513, w513) -> (reference out=w512:refnum<event-registration>, error out=w521:errorcluster)  [unwired: 1 in]
        n238 = Bundle By Name(cluster=w527, "Event Ref"=w512) -> (w522:T6)
      }
      frame "Set Parent" {
        # "Show the panel."
        # "Set the panel parent and position."
        # "Open the window as hidden, this way we can get the Hwnd but have it not be seen."
        n239 = Unbundle By Name(w549) -> ("Reposition Offset"=w550:cluster{"Left":i16, "Top":i32}, "Parent Hwnd"=w551:u32, "Current Panel.Panel Ref"=w543:refnum<vi>)
        n240 = invoke class="VI" method="FP.Open"(reference=w543, error in=w542, "Activate"=TRUE ("Activate?"), "State"=T9."Hidden") -> (reference out=w536:refnum<vi>, error out=w535:errorcluster)  [unwired: 1 in, 3 out]
        n241 = call "Get Window Handle.vi"("error in (no error)"=w535, "VI reference (calling VI)"=w536) -> ("error out"=w534:errorcluster, "HWnd Out"=w533:u32)  [unwired: 8 in]
        n242 = call "Set Parent Child Window.vi"("error in (no error)"=w534, "new parent"=w551, "child"=w533) -> ("error out"=w554:errorcluster)  [unwired: 8 in]
        n243 = call "Allow Window Resize.vi"("error in (no error)"=w554, "Allow Resize?"=TRUE ("Allow Resize"), "Hwnd"=w533) -> ("error out"=w546:errorcluster)  [unwired: 8 in]
        n244 = Bundle By Name(cluster=w549, "Current Panel.Hwnd"=w533) -> (w541:T6)
        n245 = call "Move Window (hwnd).vi"("error in (no error)"=w546, "New Position (0,0)"=w550, "HWnd"=w533) -> ("error out"=w552:errorcluster, "HWnd Out"=w547:u32)  [unwired: 6 in, 1 out]
        n246 = call "Move Window (hwnd).vi"("error in (no error)"=w552, "New Position (0,0)"=w550, "HWnd"=w547) -> ("error out"=w548:errorcluster)  [unwired: 6 in, 2 out]
        n247 = call "Redraw Window.vi"("error in (no error)"=w548, "Hwnd"=w547) -> ("error out"=w538:errorcluster)  [unwired: 9 in]
        n248 = invoke class="VI" method="FP.Open"(reference=w536, error in=w538, "Activate"=TRUE ("Activate?"), "State"=T9."Standard") -> (error out=w537:errorcluster)  [unwired: 1 in, 4 out]
      }
      frame "Load Settings" {
        # "The idea here is that you load from a file all the settings when the application exited.  Here we take that file then send that data to each UI panel element with a user event so that each UI element can load its own settings.  This will be passed as a variant because each UI element may have different needs for settings.  For example a graph may want to save the Auto Y or X settings along with the window size."
      }
      frame "Save Settings" {
        # "The idea here is that we will generate a user event for each UI panel element asking for the UI settings to save for that item.  Then we take that data as a variant and write it to a file.  We can use this information to load later by sending the same variant data back to each UI element."
      }
      frame "-----Functions-----" {
      }
      frame "Get Current Panel From VI" {
        # "Set the Current Panel to the panel with the name kept from earlier."
        n249 = Unbundle By Name(w570) -> ("New Panel VI Name"=w569:string)
        n250 = call "Panel Global Data.vi"("Method (Read All)"=Panel_Global_Methods."Read All Panels", "error in (no error)"=w566) -> ("error out"=w565:errorcluster, "All Panel Data"=w571:T4[])  [unwired: 6 in, 2 out]
        n251 = for {
          tunnel: w569 -> [w577]
          tunnel: [w574] -> w567
          tunnel: w571 -> [w574] mode=indexing
          stop <- w576 stop-if-true
          n252 = Unbundle By Name(w574) -> ("Panel VI Name"=w578:string)
          n253 = Wait (ms)(milliseconds to wait=u32 0) -> ()  [unwired: 1 out]
          n254 = Equal?(x=w578, y=w577) -> (x = y?=w576:bool)
        }
        n255 = Bundle By Name(cluster=w570, "Current Panel"=w567) -> (w568:T6)
      }
      frame "Complete Move Panel", "Prepare Move Panel" {
        n256 = Unbundle By Name(w591) -> ("Parent Hwnd"=w605:u32, "Reposition Offset"=w604:cluster{"Left":i16, "Top":i32}, "Current Panel.Panel Ref"=w590:refnum<vi>, "Current Panel.Panel VI Name"=w589:string)
        n257 = call "Panel Global Data.vi"("Method (Read All)"=Panel_Global_Methods."Read Panel Data", "error in (no error)"=w580, "Panel VI Name"=w589) -> ("error out"=w584:errorcluster, "Panel Data Out"=w587:T4)  [unwired: 5 in, 2 out]
        n258 = Unbundle By Name(w587) -> ("Hwnd"=w586:u32)
        n259 = control-ref of="Pane 2"() -> (w593:refnum<vi>)
        n260 = call "Get Child Coordinates.vi"("Child hWnd"=w586, "Parent hWnd"=w605) -> ("error out"=w585:errorcluster, "Relative"=w603:T18)  [unwired: 7 in, 1 out]
        n261 = Unbundle By Name(w603) -> ("left"=w602:i16, "top"=w601:i16)
        n262 = property on="2D Picture" class="Pict"(error in=w585) -> (error out=w582:errorcluster, "Position"=w598:T10)  [unwired: 1 in, 1 out]
        n263 = property on="Property Node" class="Pane"(reference=w593, error in=w585) -> (error out=w581:errorcluster, "Origin"=w596:T19)  [unwired: 1 out]
        n264 = Bundle("left"=w602, "top"=w601) -> (w599:cluster{"left":i16, "top":i16})  [unwired: 1 in]
        n265 = Subtract(x=w598, y=w596) -> (x-y=w597:T10)
        n266 = Add(x=w597, y=w604) -> (x+y=w594:T10)
        n267 = Add(x=w599, y=w596) -> (x+y=w600:T19)
        n268 = Subtract(x=w600, y=w604) -> (x-y=w595:cluster{i16, i32})
        n269 = case shown="\"Complete Move Panel\", Default" w592 {
          tunnel: w586 -> [w617 w643]
          tunnel: w595 -> [_ w629]
          tunnel: w594 -> [w614 _]
          tunnel: w604 -> [w613 _]
          tunnel: w590 -> [w611 w627]
          tunnel: w584 -> [w608 w624]
          tunnel: [w609 w619] -> w583
          frame "Complete Move Panel", Default {
            # "Hide the blue picture control, move the Panel VI, then show it."
            n270 = property on="2D Picture" class="Pict"(error in=w608, "Visible"=FALSE) -> (error out=w607:errorcluster)  [unwired: 1 in, 1 out]
            n271 = In Range and Coerce(upper limit=T10 {"Left"=2147483647, "Top"=2147483647}, x=w614, lower limit=w613) -> (coerced(x)=w615:T10)  [unwired: 1 out]
            n272 = call "Move Window (hwnd).vi"("error in (no error)"=w607, "New Position (0,0)"=w615, "HWnd"=w617) -> ("error out"=w610:errorcluster)  [unwired: 6 in, 2 out]
            n273 = property class="VI"(reference=w611, error in=w610, "FP.State"=T9."Standard" ("Front Panel Window:State")) -> (error out=w609:errorcluster)  [unwired: 1 out]
          }
          frame "Prepare Move Panel" {
            # "Hide the Panel VI, then replace it with a picture control that is blue and looks like the panel."
            n274 = call "Get Window Image From HWND.vi"("error in (no error)"=w624, "HWnd"=w643) -> ("error out"=w625:errorcluster, "Window Image"=w633:T20)  [unwired: 8 in]
            n275 = call <vilib>:"Unflatten Pixmap.vi"("image data"=w633) -> ("24-bit pixmap"=w642:u32[][])  [unwired: 4 in, 6 out]
            n276 = property class="VI"(reference=w627, error in=w625, "FP.State"=T9."Hidden" ("Front Panel Window:State")) -> (error out=w623:errorcluster)  [unwired: 1 out]
            n277 = Unbundle By Name(w633) -> ("Rectangle.right"=w632:i16, "Rectangle.bottom"=w631:i16)
            n278 = call "Adjust Color Image.vi"("error in (no error)"=w623, "24-bit pixmap"=w642) -> ("error out"=w622:errorcluster, "Blue Image"=w640:u32[][])  [unwired: 8 in]
            n279 = call "Empty Picture"() -> ("empty picture"=w641:picture)
            n280 = call-poly <vilib>:"Draw Unflattened Pixmap.vi"("picture"=w641, "data (RGB format)"=w640) -> ("new picture"=w637:picture)  [unwired: 7 in]
            n281 = Bundle By Name(cluster=T12 {"left"=0, "top"=0, "right"=0, "bottom"=0} ("rect"), "right"=w632, "bottom"=w631) -> (w638:T12)
            n282 = Bundle("right"=w632, "bottom"=w631) -> (w630:cluster{"right":i16, "bottom":i16})  [unwired: 1 in]
            n283 = property on="2D Picture" class="Pict"(error in=w622, "Draw Area Size"=w630) -> (error out=w621:errorcluster)  [unwired: 1 in, 1 out]
            n284 = call <vilib>:"Draw Rect.vi"("picture"=w637, "rect"=w638, "fill?(F)"=FALSE, "color(black)"=u32 22748, "pen"=T11 {"Width"=7, "Style"=enum."Solid"}) -> ("new picture"=→"2D Picture":picture)  [unwired: 4 in]
            n285 = property on="2D Picture" class="Pict"(error in=w621, "Position"=w629) -> (error out=w620:errorcluster)  [unwired: 1 in, 1 out]
            n286 = property on="2D Picture" class="Pict"(error in=w620, "Visible"=TRUE) -> (error out=w619:errorcluster)  [unwired: 1 in, 1 out]
          }
        }
        n287 = Merge Errors(w581, w582, w583) -> (w579:errorcluster)
      }
      frame "Move Panel In Range" {
        # "If the panel tried to move out of the valid range then move it back."
        n288 = Unbundle By Name(w652) -> ("Parent Hwnd"=w647:u32, "Current Panel.Hwnd"=w649:u32, "Reposition Offset"=w653:cluster{"Left":i16, "Top":i32})
        n289 = call "Get Child Coordinates.vi"("error in (no error)"=w650, "Child hWnd"=w649, "Parent hWnd"=w647) -> ("error out"=w648:errorcluster, "Relative"=w646:T18)  [unwired: 6 in, 1 out]
        n290 = call "Extract Window Origin and Size.vi"("window rect"=w646) -> ("window origin"=w645:cluster{"left":i16, "top":i16})  [unwired: 1 out]
        n291 = In Range and Coerce(upper limit=T10 {"Left"=2147483647, "Top"=2147483647}, x=w645, lower limit=w653) -> (coerced(x)=w654:T10)  [unwired: 1 out]
        n292 = call "Move Window (hwnd).vi"("error in (no error)"=w648, "New Position (0,0)"=w654, "HWnd"=w649) -> ("error out"=w651:errorcluster)  [unwired: 6 in, 2 out]
      }
      frame "Change Tabs" {
        # "Show the panels on the new tab."
        # "Hide the panels on this tab."
        n293 = Unbundle By Name(w667) -> ("Current Panel.Panel VI Name"=w670:string, "Dock Panel In New Tab"=w661:bool, "Mouse Down Move"=w657:bool, "All Panel Data"=w660:T5[], "Previous Tab"=w669:i32, "Current Tab"=w668:i32)
        n294 = Or(x=w661, y=w657) -> (x .or. y?=w664:bool)
        n295 = Index Array(array=w660, index=w669) -> (element=w677:T5)
        n296 = Index Array(array=w660, index=w668) -> (element=w673:T5)
        n297 = Unbundle By Name(w677) -> ("Panel Names"=w675:string[])
        n298 = Unbundle By Name(w673) -> ("Panel Names"=w671:string[])
        n299 = call "Show Hide Tab VIs.vi"("error in (no error)"=w663, "Front Panel State"=T9."Hidden" ("Front Panel Window:State"), "Panel Names"=w675) -> ("error out"=w674:errorcluster)  [unwired: 8 in]
        n300 = Bundle By Name(cluster=w667, "Dock Panel In New Tab"=FALSE) -> (w666:T6)
        n301 = call "Show Hide Tab VIs.vi"("error in (no error)"=w674, "Front Panel State"=T9."Standard" ("Front Panel Window:State"), "Panel Names"=w671) -> ("error out"=w659:errorcluster)  [unwired: 8 in]
        n302 = case shown="True" w664 {
          tunnel: w660 -> [_ w698]
          tunnel: w670 -> [_ w681]
          tunnel: w669 -> [_ w690]
          tunnel: w668 -> [_ w691]
          tunnel: w666 -> [w680 w689]
          tunnel: [w680 w688] -> w662
          tunnel: w659 -> [w679 w684]
          tunnel: [w679 w683] -> w658
          tunnel: w657 -> [_ w682]
          frame False {
            # "Tab changed but no panels were moved."
          }
          frame True {
            n303 = Index Array(array=w698, index=w691) -> (element=w697:T5)
            n304 = Index Array(array=w698, index=w690) -> (element=w694:T5)
            n305 = Unbundle By Name(w697) -> ("Panel Names"=w699:string[])
            n306 = Unbundle By Name(w694) -> ("Panel Names"=w701:string[])
            n307 = Search 1D Array(1D array=w701, element=w681) -> (index of element=w700:i32)  [unwired: 1 in]
            n308 = Build Array (concatenate)(w699, w681) -> (w696:string[])
            n309 = Delete From Array(array=w701, index=w700) -> (array with subset deleted=w693:string[])  [unwired: 1 in, 1 out]
            n310 = Bundle By Name(cluster=w697, "Panel Names"=w696) -> (w695:T5)
            n311 = Bundle By Name(cluster=w694, "Panel Names"=w693) -> (w692:T5)
            n312 = Build Array(w681) -> (w686:string[])
            n313 = Replace Array Subset(array=w698, new element #1=w695, index #1=w691, new element #2=w692, index #2=w690) -> (w687:T5[])
            n314 = Bundle By Name(cluster=w689, "All Panel Data"=w687) -> (w688:T6)
            n315 = case shown="False" w682 {
              tunnel: w686 -> [w705 _]
              tunnel: T9."Standard" ("Front Panel State") -> [w704 _]
              tunnel: w684 -> [w703 w706]
              tunnel: [w702 w706] -> w683
              frame False {
                n316 = call "Show Hide Tab VIs.vi"("error in (no error)"=w703, "Front Panel State"=w704, "Panel Names"=w705) -> ("error out"=w702:errorcluster)  [unwired: 8 in]
              }
              frame True {
              }
            }
          }
        }
      }
      frame "-----Development Errors-----" {
      }
      frame "Error" {
        n317 = case shown="\"Clear Error Cleanup\"" T13."Notify User Clear Error" ("Enum") {
          tunnel: w714 -> [w718 w723 w726]
          tunnel: [w717 w722 w727] -> w713
          tunnel: w711 -> [w716 w721 w724]
          tunnel: [w716 w719 w724] -> w712
          frame "Clear Error And Continue", Default {
            # "Clear error and continue"
            n318 = call <vilib>:"Clear Errors.vi"("error in (no error)"=w718) -> ("error out"=w717:errorcluster)  [unwired: 5 in, 1 out]
          }
          frame "Clear Error Cleanup" {
            # "Clear the error then run Cleanup."
            n319 = call <vilib>:"Clear Errors.vi"("error in (no error)"=w723) -> ("error out"=w722:errorcluster)  [unwired: 5 in, 1 out]
            n320 = Build Array (concatenate)(w721, "Cleanup" ("Element to Add")) -> (w719:string[])
          }
          frame "Notify User Clear Error" {
            # "Notify the user of the error then continue."
            n321 = call <vilib>:"Simple Error Handler.vi"("error in (no error)"=w726) -> ("error out"=w725:errorcluster)  [unwired: 4 in, 4 out]
            n322 = call <vilib>:"Clear Errors.vi"("error in (no error)"=w725) -> ("error out"=w727:errorcluster)  [unwired: 5 in, 1 out]
          }
        }
      }
      frame "Unhandled Case", Default {
        # "Notify the user of the unhandled case then continue."
        n323 = property class="VI"(error in=w729) -> (error out=w728:errorcluster, "Name"=w730:string)  [unwired: 1 in, 1 out]
        n324 = Format Into String(format string="Error:  Unhandled case\n\n%s\n\nIn VI %s", w731, w730) -> (resulting string=w732:string)  [unwired: 2 in, 1 out]
        n325 = One Button Dialog(message=w732) -> ()  [unwired: 1 in, 1 out]
      }
      frame "-----Exit Operations-----" {
      }
      frame "Cleanup" {
        # "When a graceful close operation is called we want to unregister for the events, then exit."
        n326 = Build Array (concatenate)(w741, string[] ["Quit Panel VIs", "Unregister Events", "Exit"]) -> (w739:string[])
      }
      frame "Quit Panel VIs" {
        # "Tell all of the Panel VIs to quit, which will tell the Child VIs to quit."
        # "Close all of the panels."
        n327 = call "Panel Global Data.vi"("Method (Read All)"=Panel_Global_Methods."Read All Panels", "error in (no error)"=w752) -> ("error out"=w753:errorcluster, "All Panel Data"=w754:T4[])  [unwired: 6 in, 2 out]
        n328 = for {
          tunnel: [w763] -> w756 mode=indexing
          tunnel: w754 -> [w762] mode=indexing
          tunnel: w753 -> [w760]
          workers-P: _ -> [_]
          n329 = Unbundle By Name(w762) -> ("Panel Ref"=w761:refnum<vi>)
          n330 = property class="VI"(reference=w761, error in=w760, "FP.State"=T9."Closed" ("Front Panel Window:State")) -> (reference out=w765:refnum<vi>, error out=w766:errorcluster)
          n331 = Wait (ms)(milliseconds to wait=u32 0) -> ()  [unwired: 1 out]
          n332 = Close Reference(reference=w765, error in (no error)=w766) -> (error out=w763:errorcluster)
        }
        n333 = Unbundle By Name(w757) -> ("Quit Event"=w751:refnum<user-event>)
        n334 = Merge Errors(w756) -> (w747:errorcluster)
        n335 = Set Variant Attribute(Variant=variant ("variant"), name="Event Name" ("Tag"), value="Quit" ("Event Name"), error in=w747) -> (Variant out=w750:variant, error out=w744:errorcluster)  [unwired: 1 out]
        n336 = Generate User Event(user event=w751, event data cluster=w750, error in=w744) -> (error out=w746:errorcluster)  [unwired: 1 in, 1 out]
      }
      frame "Unregister Events" {
        n337 = Unbundle By Name(w768) -> ("Event Ref"=w767:refnum<event-registration>)
        n338 = Unregister For Events(event registration refnum=w767, error in=w770) -> (error out=w769:errorcluster)
      }
      frame "Exit" {
        # "Code in this case will execute once on exit."
      }
    }
  }
  "error out" <- w1
